vi "onValidateExpression.vi"(8 "error in (no error)":errorcluster, 10 "Expression":string, 11 "Cron.Jenkins in":refnum<class "Cron.Jenkins.lvclass">) -> (0 "error out":errorcluster, 1 "valid?":bool, 2 "Validated Expression":string, 3 "Cron.Jenkins out":refnum<class "Cron.Jenkins.lvclass">)   [LabVIEW 2013, in "openCron.lvlib" / "Cron.Jenkins.lvclass"]
uses:
  Cron.Jenkins.lvclass
  Cron/Cron.lvclass
  <vilib>/regexp/Match Regular Expression.xnode
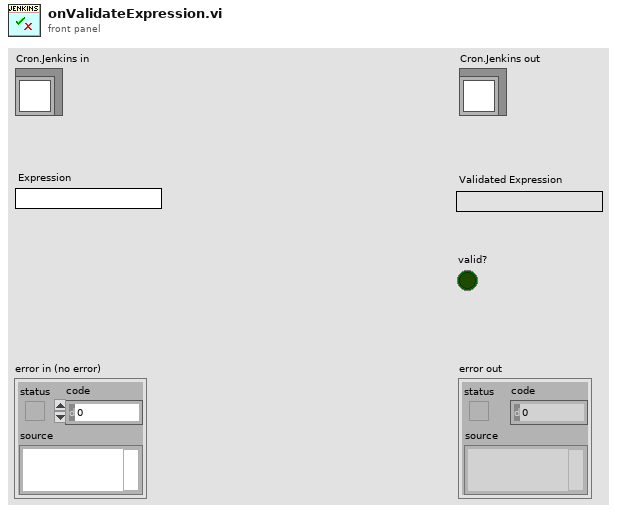
[diagram p1: front panel]
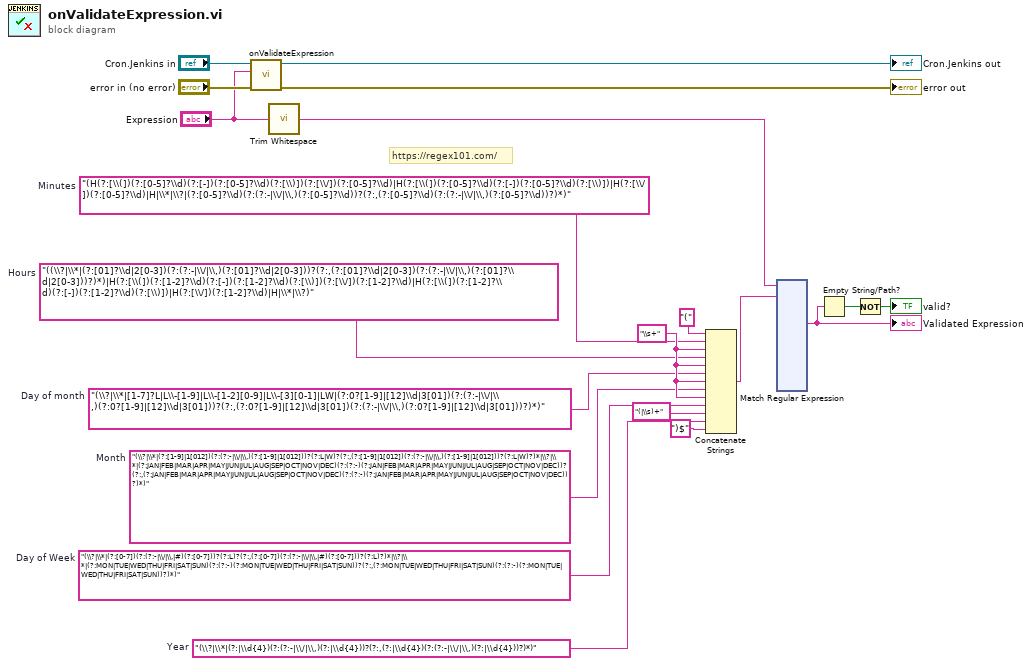
[diagram p0: block diagram]
diagram:
  w1 = "((\\?|\\*|(?:[01]?\\d|2[0-3])(?:(?:-|\\/|\\,)(?:[01]?\\d|2[0-3]))?(?:,(?:[01]?\\d|2[0-3])(?:(?:-|\\/|\\,)(?:[01]?\\d|2[0-3]))?)*)|H(?:[\\(])(?:[1-2]?\\d)(?:[-])(?:[1-2]?\\d)(?:[\\)])(?:[\\/])(?:[1-2]?\\d)|H(?:[\\(])(?:[1-2]?\\d)(?:[-])(?:[1-2]?\\d)(?:[\\)])|H(?:[\\/])(?:[1-2]?\\d)|H|\\*|\\?)"  # Hours
  w4 = "(\\?|\\*|(?:|\\d{4})(?:(?:-|\\/|\\,)(?:|\\d{4}))?(?:,(?:|\\d{4})(?:(?:-|\\/|\\,)(?:|\\d{4}))?)*)"  # Year
  w6 = "(\\?|\\*|(?:[1-9]|1[012])(?:(?:-|\\/|\\,)(?:[1-9]|1[012]))?(?:L|W)?(?:,(?:[1-9]|1[012])(?:(?:-|\\/|\\,)(?:[1-9]|1[012]))?(?:L|W)?)*|\\?|\\*|(?:JAN|FEB|MAR|APR|MAY|JUN|JUL|AUG|SEP|OCT|NOV|DEC)(?:(?:-)(?:JAN|FEB|MAR|APR|MAY|JUN|JUL|AUG|SEP|OCT|NOV|DEC))?(?:,(?:JAN|FEB|MAR|APR|MAY|JUN|JUL|AUG|SEP|OCT|NOV|DEC)(?:(?:-)(?:JAN|FEB|MAR|APR|MAY|JUN|JUL|AUG|SEP|OCT|NOV|DEC))?)*)"  # Month
  w5 = "(\\?|\\*|[1-7]?L|L\\-[1-9]|L\\-[1-2][0-9]|L\\-[3][0-1]|LW|(?:0?[1-9]|[12]\\d|3[01])(?:(?:-|\\/|\\,)(?:0?[1-9]|[12]\\d|3[01]))?(?:,(?:0?[1-9]|[12]\\d|3[01])(?:(?:-|\\/|\\,)(?:0?[1-9]|[12]\\d|3[01]))?)*)"  # Day of month
  w7 = "(\\?|\\*|(?:[0-7])(?:(?:-|\\/|\\,|#)(?:[0-7]))?(?:L)?(?:,(?:[0-7])(?:(?:-|\\/|\\,|#)(?:[0-7]))?(?:L)?)*|\\?|\\*|(?:MON|TUE|WED|THU|FRI|SAT|SUN)(?:(?:-)(?:MON|TUE|WED|THU|FRI|SAT|SUN))?(?:,(?:MON|TUE|WED|THU|FRI|SAT|SUN)(?:(?:-)(?:MON|TUE|WED|THU|FRI|SAT|SUN))?)*)"  # Day of Week
  w8 = "(H(?:[\\(])(?:[0-5]?\\d)(?:[-])(?:[0-5]?\\d)(?:[\\)])(?:[\\/])(?:[0-5]?\\d)|H(?:[\\(])(?:[0-5]?\\d)(?:[-])(?:[0-5]?\\d)(?:[\\)])|H(?:[\\/])(?:[0-5]?\\d)|H|\\*|\\?|(?:[0-5]?\\d)(?:(?:-|\\/|\\,)(?:[0-5]?\\d))?(?:,(?:[0-5]?\\d)(?:(?:-|\\/|\\,)(?:[0-5]?\\d))?)*)"  # Minutes
  w11 = "\\s+"
  # "https://regex101.com/"
  n1 = call-parent "onValidateExpression.vi"("error in (no error)"="error in (no error)", "Expression"="Expression", "Cron in"="Cron.Jenkins in") -> ("error out"=→"error out":errorcluster, "Cron out"=→"Cron.Jenkins out":refnum<class "Cron.Jenkins.lvclass">)  [unwired: 5 in, 2 out]
  n2 = call <vilib>:"Trim Whitespace.vi"("string"="Expression") -> ("trimmed string"=w15:string)  [unwired: 1 in]
  n3 = Concatenate Strings("(", w8, w11, w1, w11, w5, w11, w6, w11, w7, "(|\\s)+", w4, ")$") -> (w3:string)
  n4 = xnode "Match Regular Expression"("input string"=w15, "regular expression"=w3) -> ("submatch 1"=w14:string)  [unwired: 4 in, 13 out]
  "Validated Expression" <- w14
  n5 = Empty String/Path?(string/path=w14) -> (empty?=w13:bool)
  n6 = Not(x=w13) -> (.not. x?=→"valid?":bool)
